vi "Intake_execute.vi"() -> ()   [LabVIEW 2020]
uses:
  <vilib>/Rock Robotics/WPI/Solenoid/WPI_SolenoidValue.ctl
  Globals/Intake_Motor_global.vi
panel:
  in  "Intake_motor^2":dbl
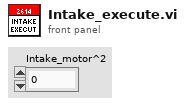
[diagram p1: front panel]
types:
  T1 = typedef "WPI_SolenoidValue.ctl" = enum16{"Off", "On", "Forward", "Reverse"}
  T2 = typedef "Intake_cluster.ctl" = cluster{"control_states":T3, "Manual_control":dbl, "Trigger?":bool, "Manual_Extend?":bool}
  T3 = typedef "Intake_control_states.ctl" = enum16{"No_Op", "Intake", "Manual"}
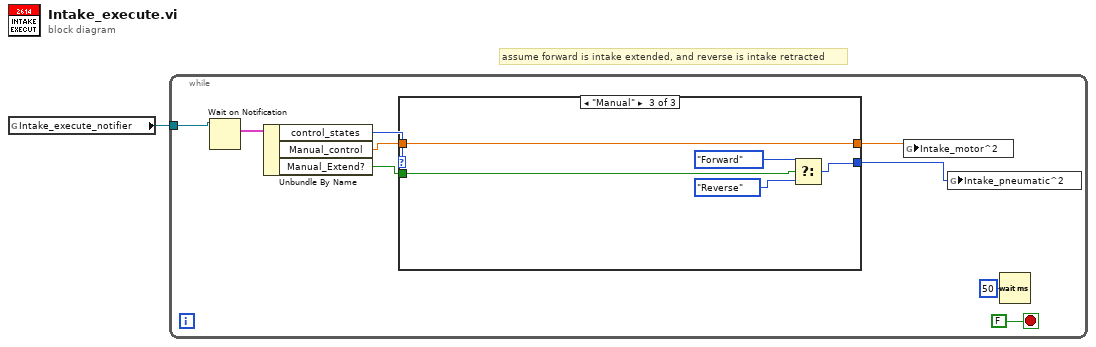
[diagram p0: block diagram]
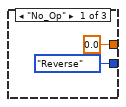
[diagram p2: hidden frame]
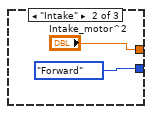
[diagram p3: hidden frame]
diagram:
  # "assume forward is intake extended, and reverse is intake retracted"
  n1 = global read "Intake_Motor_global.vi" "Intake_execute_notifier"() -> (w1:refnum<notifier>)
  n2 = while {
    tunnel: w1 -> [w10]
    stop <- FALSE stop-if-true
    n3 = Wait on Notification(notifier=w10) -> (notification=w7:T2)  [unwired: 3 in, 3 out]
    n4 = Unbundle By Name(w7) -> ("control_states"=w6:T3, "Manual_control"=w3:dbl, "Manual_Extend?"=w2:bool)
    n5 = case shown="\"Manual\"" w6 {
      tunnel: [0.0 ("Intake_motor^2") "Intake_motor^2" w19] -> w5
      tunnel: [WPI_SolenoidValue."Reverse" ("Value") WPI_SolenoidValue."Forward" ("Value") w15] -> w4
      tunnel: w3 -> [_ _ w19]
      tunnel: w2 -> [_ _ w18]
      frame "No_Op" {
      }
      frame "Intake" {
      }
      frame "Manual" {
        n6 = Select(t=WPI_SolenoidValue."Forward" ("Value"), s=w18, f=WPI_SolenoidValue."Reverse" ("Value")) -> (s? t:f=w15:T1)
      }
    }
    n7 = global write "Intake_Motor_global.vi" "Intake_motor^2"(w5) -> ()
    n8 = global write "Intake_Motor_global.vi" "Intake_pneumatic^2"(w4) -> ()
    n9 = Wait (ms)(milliseconds to wait=u32 50 ("millisecond timer value")) -> ()  [unwired: 1 out]
  }
